vi "Update.vi"(4 "TypeMap in":refnum<class "TypeMap.lvclass">, 6 "commandTimeout":i32=-1, 8 "error in (no error)":errorcluster, 10 "object in":refnum<class>, 11 "SqlMapper in":refnum<class "SqlMapper.lvclass">) -> (0 "error out":errorcluster, 1 "affectedRows":i32, 3 "SqlMapper out":refnum<class "SqlMapper.lvclass">)   [LabVIEW 2020, in "ORM.lvlib" / "TypeMap.lvclass"]
uses:
  TypeMap.lvclass
  SqlMapper/SqlMapper.lvclass
  Read Table Name.vi
  TypeMap.lvclass/TypeMap.ctl
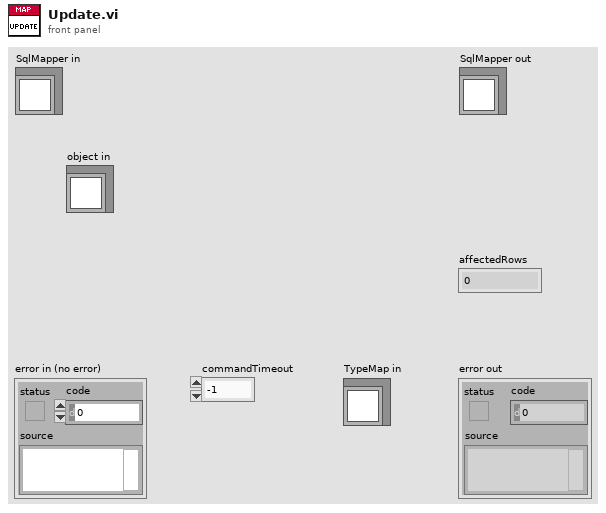
[diagram p1: front panel]
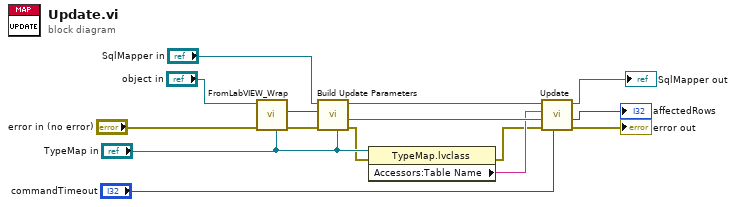
[diagram p0: block diagram]
diagram:
  n1 = call "FromLabVIEW_Wrap.vi"("TypeMap in"="TypeMap in", "error in (no error)"="error in (no error)", "object in"="object in") -> ("error out"=w10:errorcluster, "DbRow"=w9:variant)  [unwired: 7 in]
  n2 = call-dynamic "Build Update Parameters.vi"("TypeMap in"="TypeMap in", "error in (no error)"=w10, "object"=w9, "SqlMapper in"="SqlMapper in") -> ("error out"=w3:errorcluster, "DynamicParameters out"=w8:refnum<class "DynamicParameters.lvclass">, "SqlMapper out"=w6:refnum<class "SqlMapper.lvclass">)  [unwired: 5 in]
  n3 = property class="TypeMap.lvclass"(reference="TypeMap in", error in=w3) -> (error out=w2:errorcluster, "Accessors:Table Name"=w4:string)  [unwired: 1 out]
  n4 = call "Update.vi"("commandTimeout"="commandTimeout", "error in (no error)"=w2, "DynamicParameters"=w8, "TableName"=w4, "SqlMapper in"=w6) -> ("error out"=→"error out":errorcluster, "AffectedRows"=→"affectedRows":i32, "SqlMapper out"=→"SqlMapper out":refnum<class "SqlMapper.lvclass">)  [unwired: 4 in]
